vi "Get Update UE.vi"(11 "CD_Process in":refnum<class "CD_Process.lvclass">) -> (2 "Update UE":refnum<user-event>, 3 "CD_Process out":refnum<class "CD_Process.lvclass">)   [LabVIEW 2019, in "TimingDRV Engine.lvlib" / "CD_Process.lvclass"]
uses:
  CD_Process.lvclass
  TypeDefs/Update.ctl
  CD_Process.lvclass/CD_Process.ctl
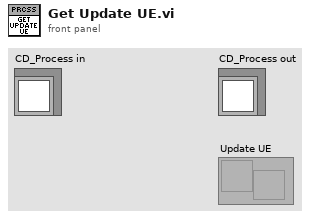
[diagram p1: front panel]
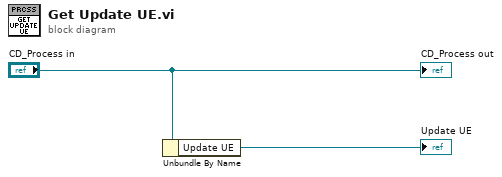
[diagram p0: block diagram]
diagram:
  n1 = Unbundle By Name("CD_Process in") -> ("Update UE"=→"Update UE":refnum<user-event>)
  "CD_Process out" <- "CD_Process in"
